vi "FV-Running_average.vi"   [LabVIEW 2020]
uses:
  FV-file_viewer.lvlib
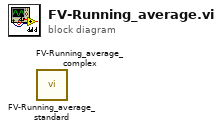
[diagram p0: block diagram]
diagram:
  n1 = call "FV-Running_average_standard.vi"() -> ()  [unwired: 11 in, 1 out]
  n2 = call "FV-Running_average_complex.vi"() -> ()  [unwired: 11 in, 1 out]
